vi "~ListboxReadValues.vi"(11 "Listbox Ref":refnum<vi>) -> (3 "Selected Values":dbl[](array[numeric]))   [LabVIEW 2017]
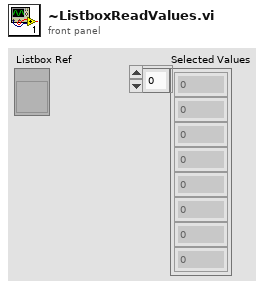
[diagram p1: front panel]
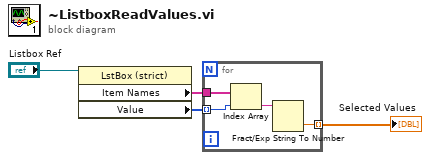
[diagram p0: block diagram]
diagram:
  n1 = property class="LstBox (strict)"(reference="Listbox Ref") -> ("Item Names"=w4:string[], "Value"=w3:i32[])  [unwired: 1 in, 2 out]
  n2 = for {
    tunnel: w4 -> [w8]
    tunnel: w3 -> [w7] mode=indexing
    tunnel: [w5] -> w2 mode=indexing
    n3 = Index Array(array=w8, index=w7) -> (element=w6:string)
    n4 = Fract/Exp String To Number(string=w6) -> (number=w5:dbl)  [unwired: 3 in, 1 out]
  }
  "Selected Values" <- w2
